vi "Read Parameters.vi"(8 "error in (no error)":errorcluster, 11 "ADAS PE Template in":refnum<class "ADAS PE Template.lvclass">) -> (0 "error out":errorcluster, 2 "Configure and Synchronize Required":bool, 3 "ADAS PE Template out":refnum<class "ADAS PE Template.lvclass">)   [LabVIEW 2020, in "ADAS PE Template.lvlib" / "ADAS PE Template.lvclass"]
doc: "<b>Read Parameters</b>\nYou do not need to edit this function.\n\nThis function loads in the configuration parameters for the plugin (for example, the file path to log to or the CAN interface name to read from)"
uses:
  ADAS PE Template.lvclass
  C:/Program Files/National Instruments/LabVIEW 2020/vi.lib/FlexLogger/SDK/PluginSDK.lvlibp/PEFClasses/SDK/Processing Element/Processing Element.lvclass
  ADAS PE Template.lvclass/ADAS PE Template.ctl
  <vilib>/FlexLogger/SDK/PluginSDK.lvlibp/PEFClasses/SDK/Processing Element/Read Alias.vi
  <vilib>/ADAS Record/Tracing/GenericEventStart.vi
  <vilib>/ADAS Record/Tracing/GenericEventStop.vi
  <vilib>/ADAS Record/Utilities/ADAS Utilities.lvlib
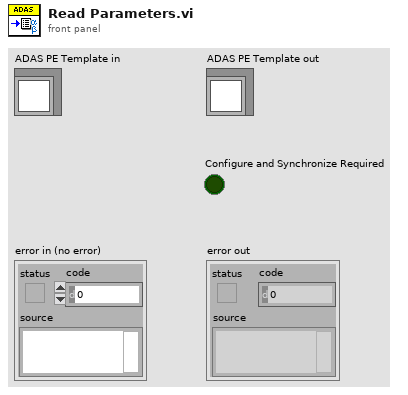
[diagram p1: front panel]
types:
  T1 = typedef "ADAS PE Template.lvlib/ADAS PE Template.lvclass/Configuration.ctl" = cluster{"Parameter1":string}
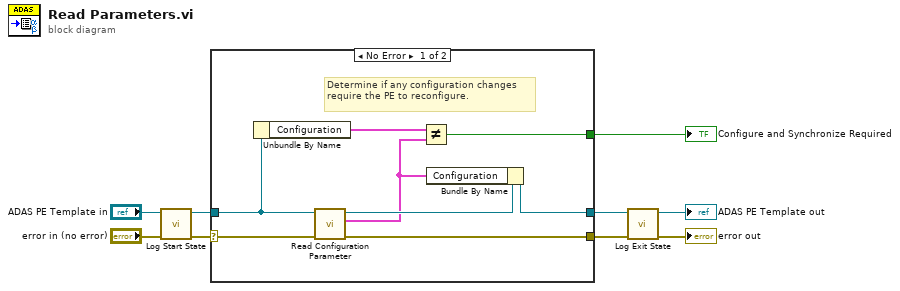
[diagram p0: block diagram]
diagram:
  n1 = call <vilib>:"Log Start State.vi"("error in (no error)"="error in (no error)", "PluginSDK.lvlibp:Processing Element.lvclass"="ADAS PE Template in") -> ("error out"=w6:errorcluster, "PluginSDK.lvlibp:Processing Element.lvclass"=w5:refnum<class "ADAS PE Template.lvclass">)  [unwired: 8 in]
  n2 = case shown="No Error" w6 {
    selector: w6 -> [w17 w19]
    tunnel: w5 -> [w13 w18]
    tunnel: [w15 w19] -> w4
    tunnel: [w14 w18] -> w2
    tunnel: [w10 _] -> w9
    frame No Error {
      # "Determine if any configuration changes require the PE to reconfigure."
      n3 = Unbundle By Name(w13) -> ("Configuration"=w11:T1)
      n4 = call "Read Configuration Parameter.vi"("error in (no error)"=w17, "ADAS PE Template in"=w13) -> ("error out"=w15:errorcluster, "Configuration"=w12:T1, "ADAS PE Template out"=w16:refnum<class "ADAS PE Template.lvclass">)  [unwired: 7 in]
      n5 = Not Equal?(x=w11, y=w12) -> (x != y?=w10:bool)
      n6 = Bundle By Name(cluster=w16, "Configuration"=w12) -> (w14:refnum<class "ADAS PE Template.lvclass">)
    }
    frame Error {
    }
  }
  "Configure and Synchronize Required" <- w9
  n7 = call <vilib>:"Log Exit State.vi"("error in (no error)"=w4, "PluginSDK.lvlibp:Processing Element.lvclass"=w2) -> ("error out"=→"error out":errorcluster, "PluginSDK.lvlibp:Processing Element.lvclass"=→"ADAS PE Template out":refnum<class "ADAS PE Template.lvclass">)  [unwired: 8 in]
